vi "PathPlanner_Cmd_AutoPathsFromCommand.vi"(11 "CommandUtil":T1) -> (0 "error out":errorcluster, 3 "Paths":T3[](array[typedef]) {"IdealStartingState"."Rotation"."SIN" format="%13.4f"; "IdealStartingState"."Rotation"."COS" format="%13.4f"; "IdealStartingState"."Rotation"."VALUE" format="%13.4f"; "PointTowardsZones"."TargetPosition"."Y" format="%14.3f"; "PointTowardsZones"."TargetPosition"."X" format="%14.3f"; "PointTowardsZones"."RotationOffset"."SIN" format="%13.4f"; "PointTowardsZones"."RotationOffset"."COS" format="%13.4f"; "PointTowardsZones"."RotationOffset"."VALUE" format="%13.4f"; "Waypoints"."nextControl"."Y" format="%14.3f"; "Waypoints"."nextControl"."X" format="%14.3f"; "Waypoints"."anchor"."Y" format="%14.3f"; "Waypoints"."anchor"."X" format="%14.3f"; "Waypoints"."prevControl"."Y" format="%14.3f"; "Waypoints"."prevControl"."X" format="%14.3f"; "AllPoints"."RotationTarget"."rotation"."SIN" format="%13.4f"; "AllPoints"."RotationTarget"."rotation"."COS" format="%13.4f"; "AllPoints"."RotationTarget"."rotation"."VALUE" format="%13.4f"; "AllPoints"."Position"."Y" format="%14.3f"; "AllPoints"."Position"."X" format="%14.3f"; "GoalEndState"."Rotation"."SIN" format="%13.4f"; "GoalEndState"."Rotation"."COS" format="%13.4f"; "GoalEndState"."Rotation"."VALUE" format="%13.4f"; "RotationTargets"."rotation"."SIN" format="%13.4f"; "RotationTargets"."rotation"."COS" format="%13.4f"; "RotationTargets"."rotation"."VALUE" format="%13.4f"})   [LabVIEW 2019, in "PathPlanner24.lvlib"]
doc: "DOCUMENTATION IS NOT COMPLETE.\n \nPack controller tuning configuration for Path Planner Holonomic Drive Controller.\n\nInputs:\n - X PID Tuning - cluster - Input from PACK PROF PID VI\n - Y PID Tuning - cluster - Input from PACK PROF PID VI\n - thetaController - cluster - A profiled PID controller to respond to error in angle.\n - Max Wheel Speed M/.S - double - Maximum wheel speed (M/S)\n - DriveBaseRadius - double - The radius of the drive base in meters. For swerve drive, this is the\n distance from the center of the robot to the furthest module. For \n mecanum, this is the drive base width / 2\n - X Tolerance - double - X tolerance for calculating At Reference (Meters) (Optional. Default: 0.0762 )\n - Y Tolerance - double - Y tolerance for calculating At Reference (Meters) (Optional. Default: 0.0762 )\n - Rotation Tolerance - double - Rotation tolerance for calculating At Reference (Degrees) (Optional. Default: 0.0)873)\n\nOutputs:\n -- PathPlannerHolCtrlConfig -- cluster - packed controller configuration."
uses:
  PathPlanner24.lvlib
  TypeDef/PathPlannerPath.ctl
  TypeDef/PathPlannerRotationTarget.ctl
  <vilib>/Rock Robotics/WPI/ThirdParty/JAS_Junk/TrajLib/TypeDef/ROTATION2D.ctl
  TypeDef/PathPlannerConstraintsZone.ctl
  TypeDef/PathPlannerPathConstraints.ctl
  TypeDef/PathPlannerEventMarker.ctl
  TypeDef/PathPlannerCommandUtil.ctl
  ENum/PathPlanner_CommandUtilType_ENUM.ctl
  TypeDef/PathPlannerGoalEndState.ctl
  TypeDef/PathPlannerPathPoint.ctl
  <vilib>/Rock Robotics/WPI/ThirdParty/JAS_Junk/TrajLib/TypeDef/TRANSLATION2D.ctl
  TypeDef/PathPlannerWaypoint.ctl
  TypeDef/PathPlannerPointTowardsZone.ctl
  TypeDef/PathPlannerIdealStartingState.ctl
  <vilib>/Rock Robotics/WPI/ThirdParty/JAS_Junk/TrajLib/Trajectory_Library.lvlib
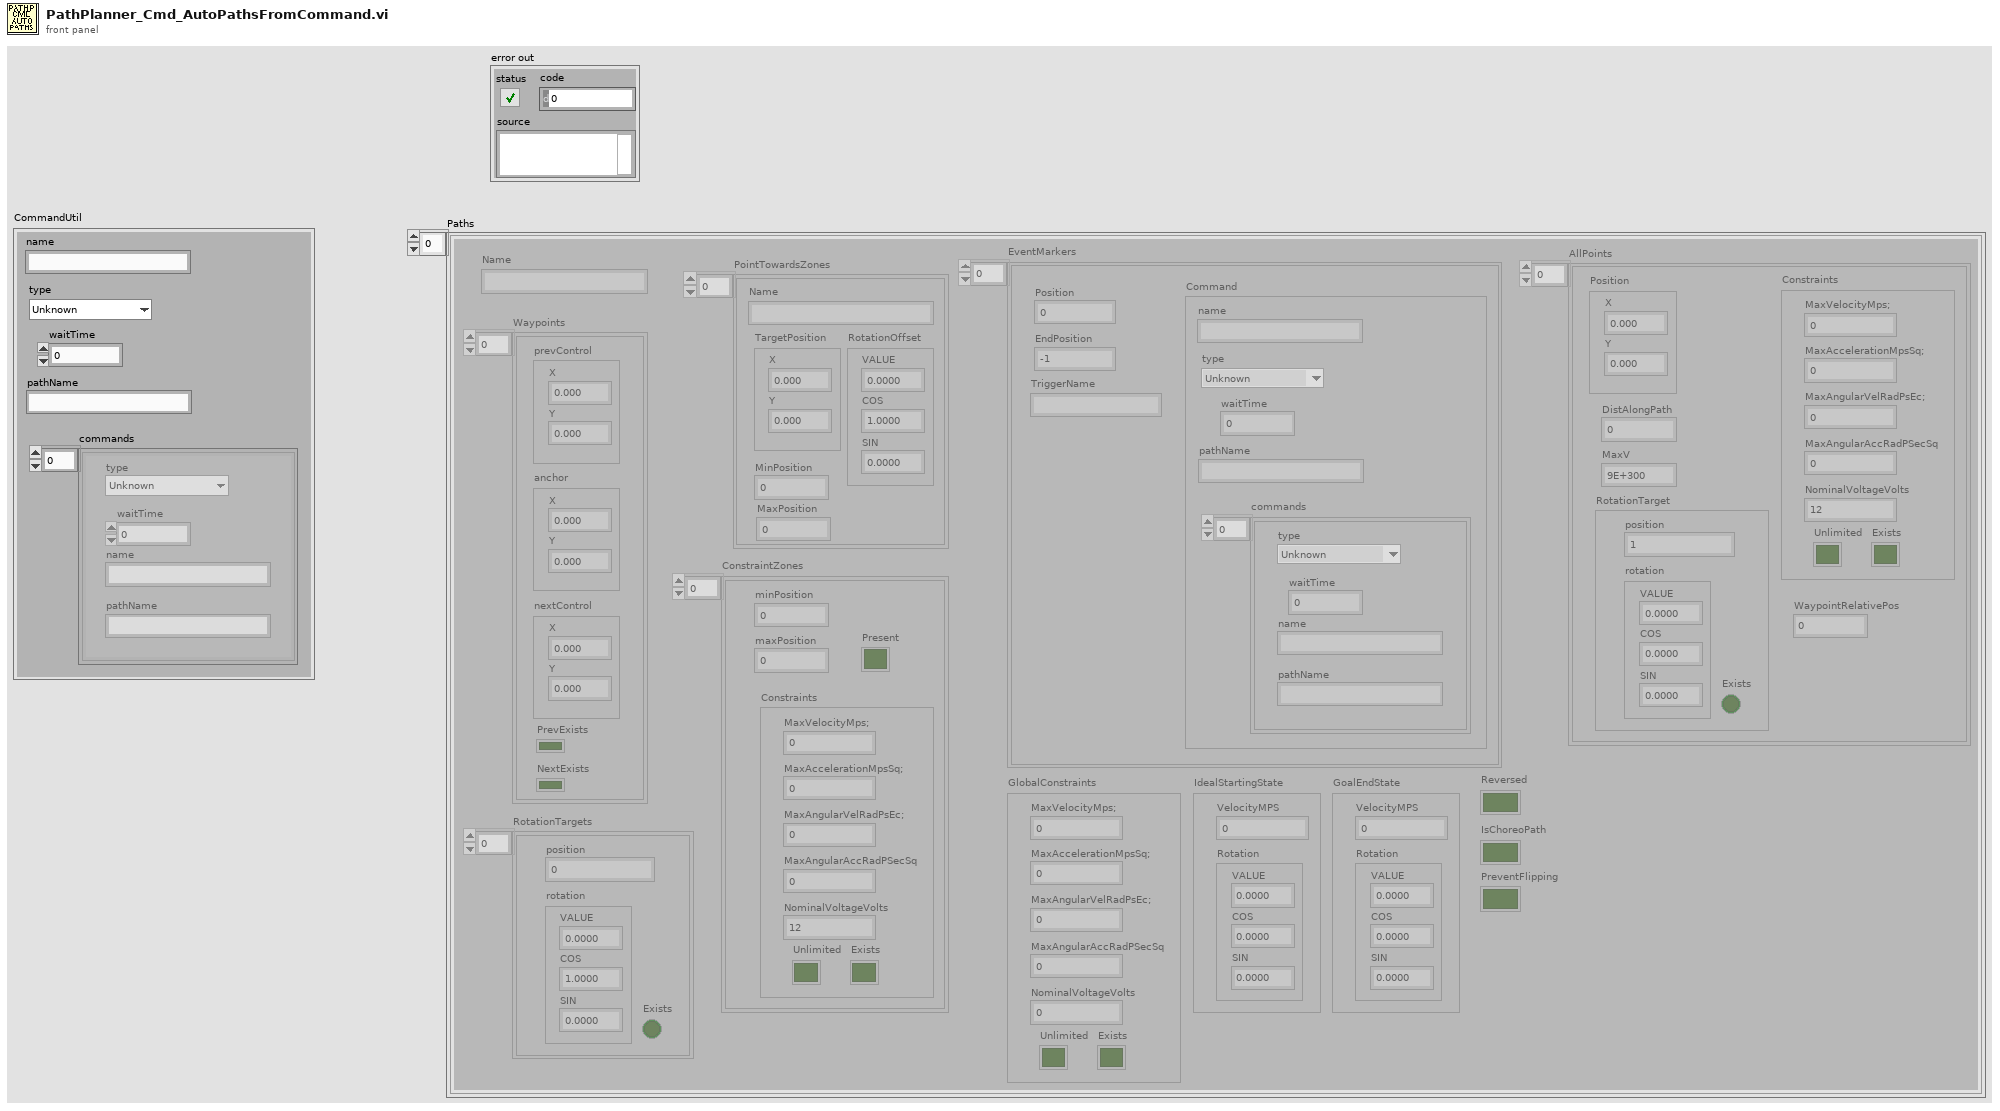
[diagram p1: front panel]
types:
  T1 = typedef "PathPlanner24.lvlib/PathPlannerCommandUtil.ctl" = cluster{"waitTime":dbl, "name":string, "pathName":string, "commands":cluster{"type":T2, "waitTime":dbl, "name":string, "pathName":string}[], "type":T2}
  T2 = typedef "PathPlanner24.lvlib/PathPlanner_CommandUtilType_ENUM.ctl" = enum16{"Unknown", "Wait", "Named", "Path", "Sequential", "Parallel", "Race", "Deadline"}
  T3 = typedef "PathPlanner24.lvlib/PathPlannerPath.ctl" = cluster{"Reversed":bool, "RotationTargets":T4[], "ConstraintZones":T6[], "EventMarkers":T8[], "GlobalConstraints":T7, "GoalEndState":T9, "AllPoints":T10[], "Name":string, "Waypoints":T12[], "PointTowardsZones":T13[], "IdealStartingState":T14, "IsChoreoPath":bool, "PreventFlipping":bool}
  T4 = typedef "PathPlanner24.lvlib/PathPlannerRotationTarget.ctl" = cluster{"position":dbl, "rotation":T5, "Exists":bool}
  T5 = typedef "Trajectory_Library.lvlib/ROTATION2D.ctl" = cluster{"VALUE":dbl, "COS":dbl, "SIN":dbl}
  T6 = typedef "PathPlanner24.lvlib/PathPlannerConstraintsZone.ctl" = cluster{"minPosition":dbl, "maxPosition":dbl, "Constraints":T7, "Present":bool}
  T7 = typedef "PathPlanner24.lvlib/PathPlannerPathConstraints.ctl" = cluster{"MaxVelocityMps;":dbl, "MaxAccelerationMpsSq;":dbl, "MaxAngularVelRadPsEc;":dbl, "MaxAngularAccRadPSecSq":dbl, "Exists":bool, "Unlimited":bool, "NominalVoltageVolts":dbl}
  T8 = typedef "PathPlanner24.lvlib/PathPlannerEventMarker.ctl" = cluster{"Position":dbl, "Command":T1, "TriggerName":string, "EndPosition":dbl}
  T9 = typedef "PathPlanner24.lvlib/PathPlannerGoalEndState.ctl" = cluster{"VelocityMPS":dbl, "Rotation":T5}
  T10 = typedef "PathPlanner24.lvlib/PathPlannerPathPoint.ctl" = cluster{"Position":T11, "DistAlongPath":dbl, "MaxV":dbl, "Constraints":T7, "RotationTarget":T4, "WaypointRelativePos":dbl}
  T11 = typedef "Trajectory_Library.lvlib/TRANSLATION2D.ctl" = cluster{"X":dbl, "Y":dbl}
  T12 = typedef "PathPlanner24.lvlib/PathPlannerWaypoint.ctl" = cluster{"prevControl":T11, "anchor":T11, "nextControl":T11, "PrevExists":bool, "NextExists":bool}
  T13 = typedef "PathPlanner24.lvlib/PathPlannerPointTowardsZone.ctl" = cluster{"RotationOffset":T5, "Name":string, "TargetPosition":T11, "MinPosition":dbl, "MaxPosition":dbl}
  T14 = typedef "PathPlanner24.lvlib/PathPlannerIdealStartingState.ctl" = cluster{"VelocityMPS":dbl, "Rotation":T5}
  T15 = cluster{"type":T2, "waitTime":dbl, "name":string, "pathName":string}[]
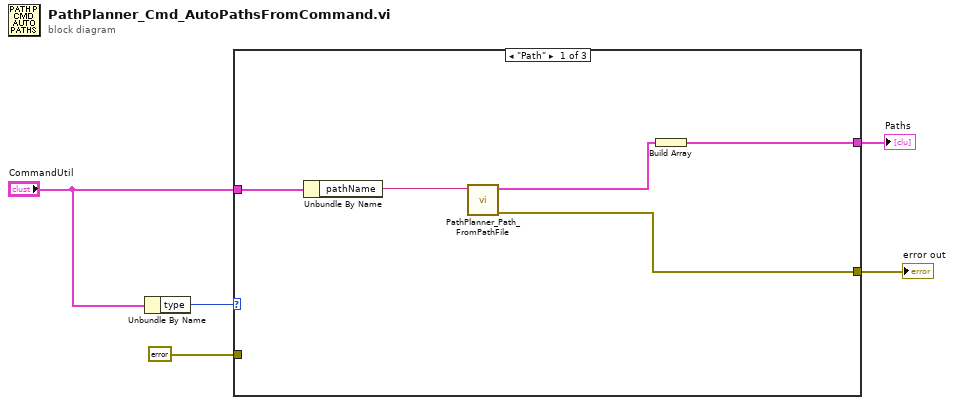
[diagram p0: block diagram]
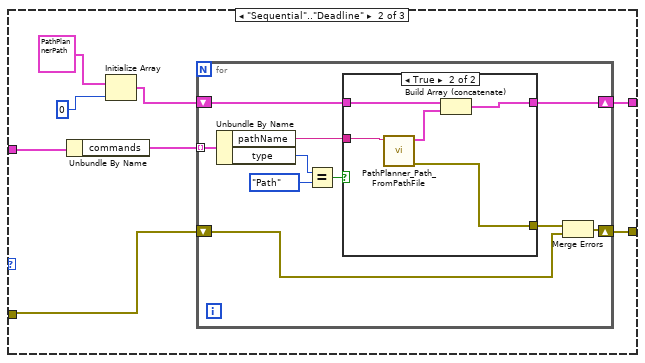
[diagram p2: hidden frame]
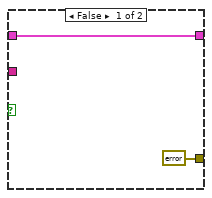
[diagram p3: hidden frame]
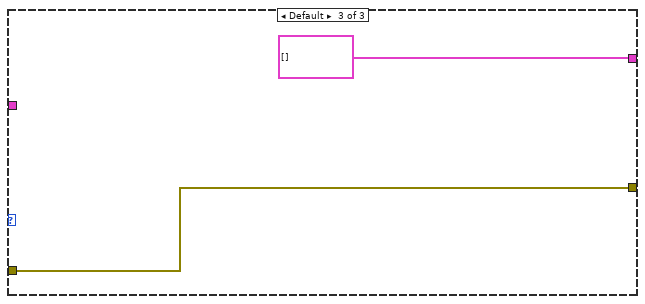
[diagram p4: hidden frame]
diagram:
  n1 = Unbundle By Name("CommandUtil") -> ("type"=w5:T2)
  n2 = case shown="\"Path\"" w5 {
    tunnel: "CommandUtil" -> [w9 w18 _]
    tunnel: [w8 w16 T3[] []] -> w4
    tunnel: errorcluster {"status"=FALSE, "code"=0, "source"=""} ("error out") -> [_ w12 w36]
    tunnel: [w6 w11 w36] -> w1
    frame "Path" {
      n3 = Unbundle By Name(w9) -> ("pathName"=w10:string)
      n4 = call "PathPlanner_Path_FromPathFile.vi"("FileName"=w10) -> ("error out"=w6:errorcluster, "PathPlannerPath"=w7:T3)  [unwired: 7 in, 2 out]
      n5 = Build Array(w7) -> (w8:T3[])
    }
    frame "Sequential".."Deadline" {
      n6 = Unbundle By Name(w18) -> ("commands"=w17:T15)
      n7 = Initialize Array(T3 {"Reversed"=FALSE, "RotationTargets"=[], "ConstraintZones"=[], "EventMarkers"=[], "GlobalConstraints"={"MaxVelocityMps;"=0.0, "MaxAccelerationMpsSq;"=0.0, "MaxAngularVelRadPsEc;"=0.0, "MaxAngularAccRadPSecSq"=0.0, "Exists"=FALSE, "Unlimited"=FALSE, "NominalVoltageVolts"=12.0}, "GoalEndState"={"VelocityMPS"=0.0, "Rotation"={"VALUE"=0.0, "COS"=1.0, "SIN"=0.0}}, "AllPoints"=[], "Name"="", "Waypoints"=[], "PointTowardsZones"=[], "IdealStartingState"={"VelocityMPS"=0.0, "Rotation"={"VALUE"=0.0, "COS"=1.0, "SIN"=0.0}}, "IsChoreoPath"=FALSE, "PreventFlipping"=FALSE} ("PathPlannerPath"), 0 ("dimension size")) -> (w13:T3[])
      n8 = for {
        tunnel: w17 -> [w28] mode=indexing
        shift-right: [w22] -> w16
        shift-left: w13 -> [w23]
        shift-right: [w19] -> w11
        shift-left: w12 -> [w20]
        n9 = Unbundle By Name(w28) -> ("pathName"=w24:string, "type"=w27:T2)
        n10 = Equal?(x=w27, y=PathPlanner_CommandUtilType_ENUM."Path") -> (x = y?=w25:bool)
        n11 = case shown="True" w25 {
          tunnel: w24 -> [_ w35]
          tunnel: w23 -> [w30 w34]
          tunnel: [w30 w32] -> w22
          tunnel: [errorcluster {"status"=FALSE, "code"=0, "source"=""} ("error out") w31] -> w21
          frame False {
          }
          frame True {
            n12 = call "PathPlanner_Path_FromPathFile.vi"("FileName"=w35) -> ("error out"=w31:errorcluster, "PathPlannerPath"=w33:T3)  [unwired: 7 in, 2 out]
            n13 = Build Array (concatenate)(w34, w33) -> (w32:T3[])
          }
        }
        n14 = Merge Errors(w21, w20) -> (w19:errorcluster)
      }
    }
    frame Default {
    }
  }
  "Paths" <- w4
  "error out" <- w1
